vi "Compute Shared Key.vi"(9 "GUID":string, 10 "SecretKey":string) -> (2 "Shared Key":string)   [LabVIEW 2021, in "smo.lvlib" / "Attribute.Owner.lvclass"]
uses:
  Attribute.Owner.lvclass
  Attribute.Owner.lvclass/Attribute.Owner.ctl
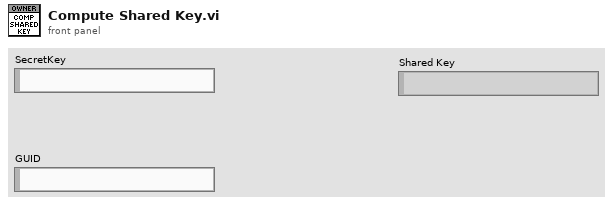
[diagram p1: front panel]
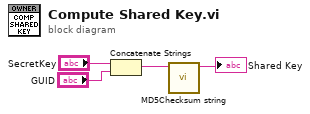
[diagram p0: block diagram]
diagram:
  n1 = Concatenate Strings("SecretKey", "GUID") -> (w2:string)
  n2 = call <vilib>:"MD5Checksum string.vi"("Message String"=w2) -> ("MD5 message-digest"=→"Shared Key":string)  [unwired: 10 in]
